vi "Gyro Auton.vi"   [LabVIEW 2015]
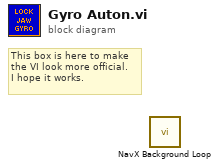
[diagram p0: block diagram]
diagram:
  # "This box is here to make\nthe VI look more official.\nI hope it works."
  n1 = call "NavX Background Loop.vi"() -> ()  [unwired: 12 in]
